vi "fgv_Triggers Output Setup.vi"(6 "Which file? (User profile.ini)":T3=enum."Loaded User profile.ini", 8 "error in (no error)":errorcluster, 9 "General trigger settings":T1={"Trigger 1 function"=enum."Encoder trigger", "Triggers loop clock (MHz)"=80.0} {"Triggers loop clock (MHz)" format="%#_13g"}, 10 "Function":T6, 11 "Triggers output setup":T4 {"Pulse width (us)" min=10 max=5000 step=1 format="%.0fµs"}) -> (0 "error out":errorcluster, 1 "General trigger settings":T1={"Trigger 1 function"=enum."Encoder trigger", "Triggers loop clock (MHz)"=80.0} {"Triggers loop clock (MHz)" format="%#_13g"}, 3 "Triggers output setup":T4 {"Pulse width (us)" min=10 max=5000 step=1 format="%.0fµs"})   [LabVIEW 2020]
uses:
  Typedefs/HW config states enum.ctl
  Peripherals Control/Triggers/Typedefs/Triggers output setup.ctl
  Peripherals Control/Triggers/Typedefs/Trigger setup element cluster.ctl
  Typedefs/Which path.ctl
  Peripherals Control/Triggers/Typedefs/General trigger settings cluster.ctl
  Typedefs/Trigger 1 selector enum.ctl
  Typedefs/Save-Load enum.ctl
  General Globals.vi
panel:
  # "FUNCTIONAL GLOBAL"
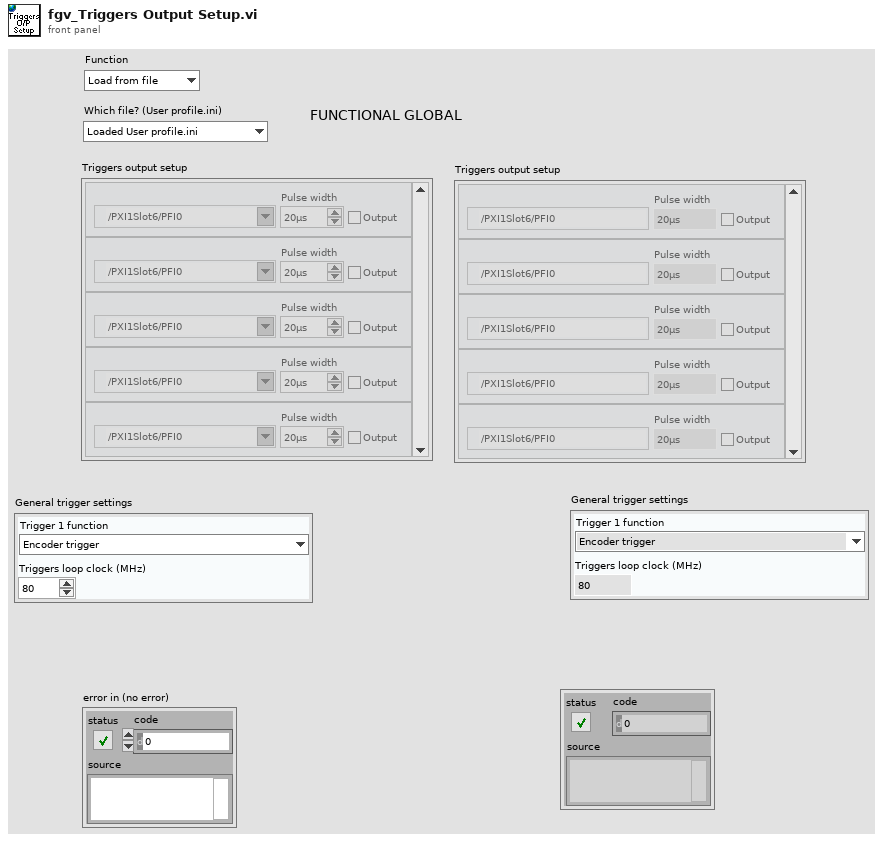
[diagram p1: front panel]
types:
  T1 = typedef "General trigger settings cluster.ctl" = cluster{"Trigger 1 function":T2, "Triggers loop clock (MHz)":dbl}
  T2 = typedef "Trigger 1 selector enum.ctl" = enum16{"Encoder trigger", "Line trigger", "Control system's ref frame acknowledgement"}
  T3 = typedef "Which path.ctl" = enum16{"Configuration Files", "Calibration Files", "Images", "Setup.ini", "Loaded User profile.ini", "User's-Previous session.ini", "New user profile.ini", "Selected User profile.ini", "User profiles folder", "Power meter scaling.txt", "FOV Cal.ini", "Calibration.ini"}
  T4 = typedef "Triggers output setup.ctl" = T5[]
  T5 = typedef "Trigger setup element cluster.ctl" = cluster{"Name":string, "Output?":bool, "Output terminal":tag, "PXI backplane line":tag, "Pulse width (us)":u16}
  T6 = typedef "HW config states enum.ctl" = enum16{"Load from file", "Save to file", "Save backup", "Write all", "Read all", "Write XY stage settings", "Write DAQ FPGA settings", "Write Control FPGA settings", "Write Phys Channels", "Write System Config", "Write HW Config", "Save System Config", "Save HW Config", "Clear", "Compare from file"}
  T7 = typedef "Save-Load enum.ctl" = enum16{"Save to file", "Load from file", "Compare from file", "Save Backup"}
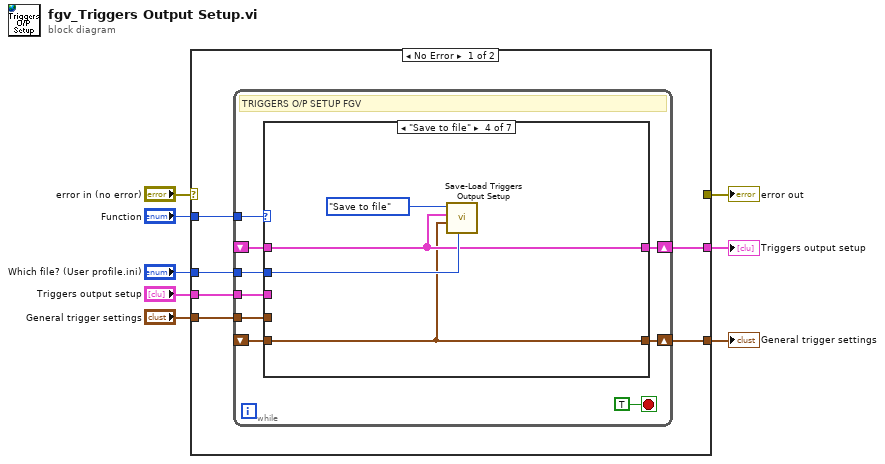
[diagram p0: block diagram]
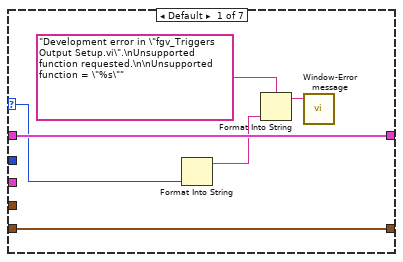
[diagram p2: hidden frame]
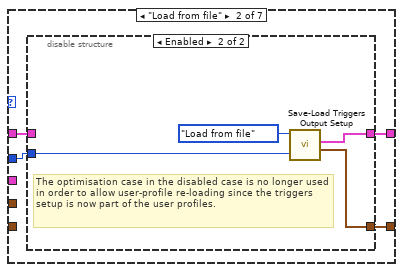
[diagram p3: hidden frame]
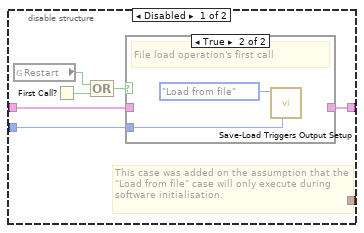
[diagram p4: hidden frame]
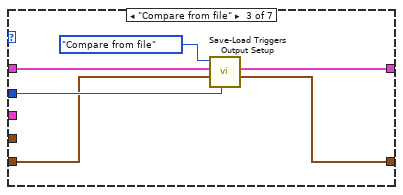
[diagram p6: hidden frame]
diagram:
  n1 = case shown="No Error" "error in (no error)" {
    selector: "error in (no error)" -> [_ w61]
    tunnel: [_ w61] -> w7
    tunnel: "Function" -> [w14 _]
    tunnel: "Triggers output setup" -> [w13 _]
    tunnel: [w12 _] -> w4
    tunnel: "Which file? (User profile.ini)" -> [w11 _]
    tunnel: "General trigger settings" -> [w10 _]
    tunnel: [w9 _] -> w1
    frame No Error {
      n2 = while {
        tunnel: w14 -> [w23]
        shift-right: [w21] -> w12
        shift-left: _ -> [w19]
        tunnel: w13 -> [w20]
        tunnel: w11 -> [w18]
        tunnel: w10 -> [w17]
        shift-right: [w16] -> w9
        shift-left: _ -> [w15]
        stop <- TRUE stop-if-true
        # "TRIGGERS O/P SETUP FGV"
        n3 = case shown="\"Save to file\"" w23 {
          selector: w23 -> [w28 _ _ _ _ _ _]
          tunnel: [w29 w33 w50 w54 w58 w60 _] -> w21
          tunnel: w20 -> [_ _ _ _ w58 _ _]
          tunnel: w19 -> [w29 w32 w49 w54 _ w60 _]
          tunnel: w18 -> [_ w31 w52 w55 _ _ _]
          tunnel: w17 -> [_ _ _ _ w57 _ _]
          tunnel: [w24 w30 w48 w53 w57 w59 _] -> w16
          tunnel: w15 -> [w24 _ w47 w53 _ w59 _]
          frame Default {
            n4 = Format Into String(w28) -> (resulting string=w26:string)  [unwired: 3 in, 1 out]
            n5 = Format Into String(format string="Development error in \"fgv_Triggers Output Setup.vi\".\nUnsupported function requested.\n\nUnsupported function = \"%s\"" ("Message"), w26) -> (resulting string=w25:string)  [unwired: 2 in, 1 out]
            n6 = call "Window-Error message.vi"("Message"=w25) -> ()  [unwired: 10 in, 1 out]
          }
          frame "Load from file" {
            n7 = disable-structure shown="Enabled" {
              disable-tunnel: [w39 w44] -> w33
              disable-tunnel: w32 -> [w38 _]
              disable-tunnel: w31 -> [w34 w46]
              disable-tunnel: [_ w43] -> w30
              frame Disabled {
                # "This case was added on the assumption that the \"Load from file\" case will only execute during software initialisation."
                n8 = global read "General Globals.vi" "Restart"() -> (w36:bool)
                n9 = First Call?() -> (First Call?: T/F=w37:bool)
                n10 = Compound Arithmetic op=OR(w36, w37) -> (w35:bool)
                n11 = case shown="True" w35 {
                  tunnel: [w40 _] -> w39
                  tunnel: w38 -> [w40 _]
                  tunnel: w34 -> [_ w41]
                  frame False {
                    # "Already loaded"
                  }
                  frame True {
                    # "File load operation's first call"
                    n12 = call "Save-Load Triggers Output Setup.vi"("Which file? (User profile.ini)"=w41, "Function"=Save-Load_enum."Load from file") -> ()  [unwired: 7 in, 3 out]
                  }
                }
              }
              frame Enabled {
                # "The optimisation case in the disabled case is no longer used in order to allow user-profile re-loading since the triggers setup is now part of the user profiles."
                n13 = call "Save-Load Triggers Output Setup.vi"("Which file? (User profile.ini)"=w46, "Function"=Save-Load_enum."Load from file") -> ("General trigger settings"=w43:T1, "Triggers output setup"=w44:T4)  [unwired: 7 in, 1 out]
              }
            }
          }
          frame "Compare from file" {
            n14 = call "Save-Load Triggers Output Setup.vi"("Which file? (User profile.ini)"=w52, "General trigger settings"=w47, "Triggers output setup to save"=w49, "Function"=Save-Load_enum."Compare from file") -> ("General trigger settings"=w48:T1, "Triggers output setup"=w50:T4)  [unwired: 5 in, 1 out]
          }
          frame "Save to file" {
            n15 = call "Save-Load Triggers Output Setup.vi"("Which file? (User profile.ini)"=w55, "General trigger settings"=w53, "Triggers output setup to save"=w54, "Function"=Save-Load_enum."Save to file") -> ()  [unwired: 5 in, 3 out]
          }
          frame "Write all" {
          }
          frame "Read all" {
          }
          frame "Clear" {
          }
        }
      }
    }
    frame Error {
    }
  }
  "error out" <- w7
  "Triggers output setup" <- w4
  "General trigger settings" <- w1
